vi "Enqueue.vi"(7 "Opposite?":bool, 8 "error in (no error)":errorcluster, 10 "Command":string, 11 "name (unnamed)":string) -> (0 "error out":errorcluster)   [LabVIEW 2011]
doc: "Enqueues a state/command on a named string-based queue.\n\n\nVersion 1.0 - 02/13/2013\n\nPhaeron, Inc.\nwww.phaeron.com\ninfo@phaeron.com"
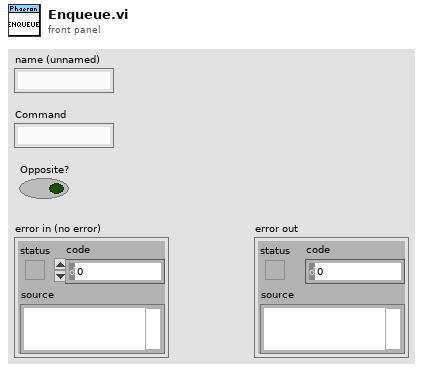
[diagram p1: front panel]
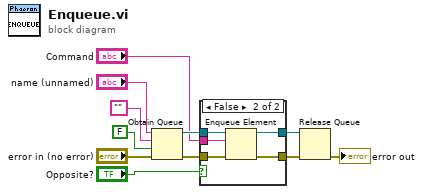
[diagram p0: block diagram]
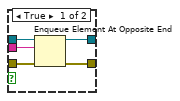
[diagram p2: hidden frame]
diagram:
  n1 = Obtain Queue(name (unnamed)="name (unnamed)", element data type="", create if not found? (T)=FALSE, error in (no error)="error in (no error)") -> (queue out=w10:refnum<queue>, error out=w8:errorcluster)  [unwired: 1 in, 1 out]
  n2 = case shown="False" "Opposite?" {
    tunnel: [w16 w21] -> w11
    tunnel: w10 -> [w15 w20]
    tunnel: [w14 w19] -> w9
    tunnel: w8 -> [w13 w18]
    tunnel: "Command" -> [w12 w17]
    frame True {
      n3 = Enqueue Element At Opposite End(queue=w15, element=w12, error in (no error)=w13) -> (queue out=w16:refnum<queue>, error out=w14:errorcluster)  [unwired: 1 in, 1 out]
    }
    frame False {
      n4 = Enqueue Element(queue=w20, element=w17, error in (no error)=w18) -> (queue out=w21:refnum<queue>, error out=w19:errorcluster)  [unwired: 1 in, 1 out]
    }
  }
  n5 = Release Queue(queue=w11, error in (no error)=w9) -> (error out=→"error out":errorcluster)  [unwired: 1 in, 2 out]
